vi "Two Circles Optimization_Func.vi"(9 "output selector":T1, 10 "data":variant, 11 "X":dbl[](array[numeric])) -> (0 "error out":errorcluster, 1 "Inequality Constraints":dbl[](array[numeric]), 2 "Equality Constraints":dbl[](array[numeric]), 3 "Objective Functions":dbl[](array[numeric]))   [LabVIEW 2023]
doc: "Two Circles Optimization function."
uses:
  <vilib>/gmath/NumericalOptimization/cno_output select.ctl
  <vilib>/gmath/NI_Gmath.lvlib
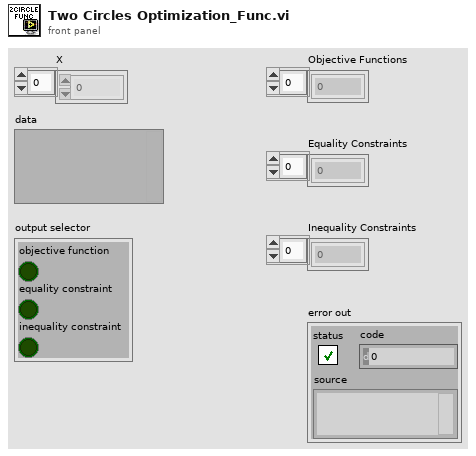
[diagram p1: front panel]
types:
  T1 = typedef "NI_Gmath.lvlib/cno_output select.ctl" = cluster{"objective function":bool, "equality constraint":bool, "inequality constraint":bool}
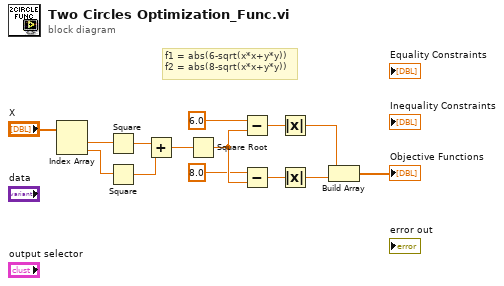
[diagram p0: block diagram]
diagram:
  # "f1 = abs(6-sqrt(x*x+y*y))\nf2 = abs(8-sqrt(x*x+y*y))"
  n1 = Index Array(array="X") -> (element #1=w14:dbl, element #2=w13:dbl)  [unwired: 2 in]
  n2 = Square(x=w14) -> (x^2=w12:dbl)
  n3 = Square(x=w13) -> (x^2=w11:dbl)
  n4 = Add(x=w12, y=w11) -> (x+y=w10:dbl)
  n5 = Square Root(x=w10) -> (sqrt(x)=w9:dbl)
  n6 = Subtract(x=6.0, y=w9) -> (x-y=w5:dbl)
  n7 = Subtract(x=8.0, y=w9) -> (x-y=w6:dbl)
  n8 = Absolute Value(x=w5) -> (abs(x)=w4:dbl)
  n9 = Absolute Value(x=w6) -> (abs(x)=w3:dbl)
  n10 = Build Array(w4, w3) -> (→"Objective Functions":dbl[])
